vi "Init.vi"(4 "Base Path":path, 6 "Template Name":string, 8 "Project:Active Project":refnum<vi>, 9 "Application Instance":refnum<vi>, 10 "Name":string, 11 "Msg Script Strategy in":refnum<class "Msg Script Strategy.lvclass">) -> (3 "Msg Script Strategy out":refnum<class "Msg Script Strategy.lvclass">)   [LabVIEW 2021, in "_Create From Template.lvlib" / "Script Strategy.lvlib" / "Msg Script Strategy.lvclass"]
uses:
  Msg Script Strategy.lvclass
  Msg Script Strategy.lvclass/Msg Script Strategy.ctl
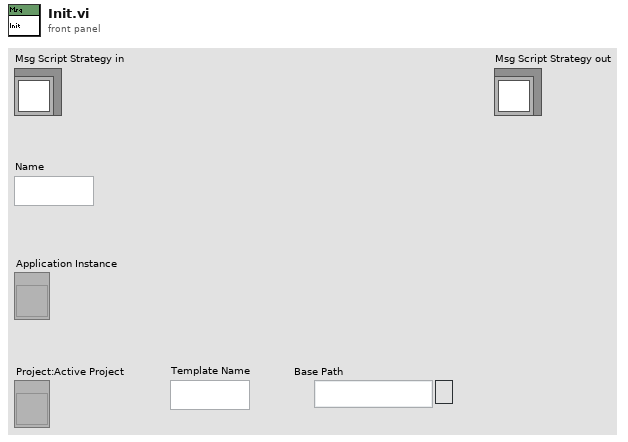
[diagram p1: front panel]
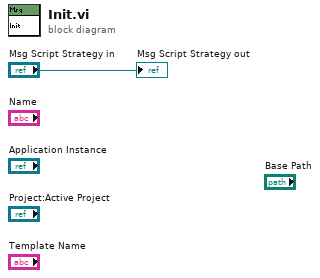
[diagram p0: block diagram]
diagram:
  "Msg Script Strategy out" <- "Msg Script Strategy in"
